vi "main.vi"() -> ()   [LabVIEW 2022 SP3]
uses:
  controls/State_control.ctl
  controls/Data.ctl
  <vilib>/Analysis/baseanly.llb/Mean (DBL).vi
  <vilib>/Utility/TDMS File Viewer/NI_TDMS File Viewer.lvlib
  <vilib>/Analysis/NI_AALBase.lvlib
panel:
  out "Prumerna teplota":dbl(graph)=53.18446
  out "Rozsah error":bool=TRUE
  out "Real-Time mereni":string[][](table)
  out "Prumerovane hodnoty":string[][](table)
  in  "vzorky/s":enum16{"Slow - 0.25 vz/s", "Fast - 12 vz/s"}(ring)=enum."Fast - 12 vz/s"
  in  "Pocet vz.":u16=20
  in  "Prumerovani":u16=10 min=1 max=20 step=1
  in  "Stop":bool
  in  "Koeficient termistoru [1/°C]":dbl=0.00385
  in  "Nazev souboru .tdms":path
  out "IDN Agilent 34450A":string
  out "Proud":dbl(graph)=0.489824809
  out "Napeti":dbl(graph)=53.18446
  out "IDN GPD-3303S":string
  in  "GPD-3303S":refnum<visa-resource-name>="zdroj"
  in  "Konec":bool
  in  "Start meas":bool
  out "IDN Agilent 34401A":string
  in  "Agilent 34401A":refnum<visa-resource-name>="01A"
  in  "Agilent 34450A":refnum<visa-resource-name>="50A"
  out "Stav":T1
  out "Ramecek":bool
  # "Kanaly"
  # "Parametry mereni"
  # "Uzivateli je doporuceno hodnoty zaokrouhlit podle platych pravidel"
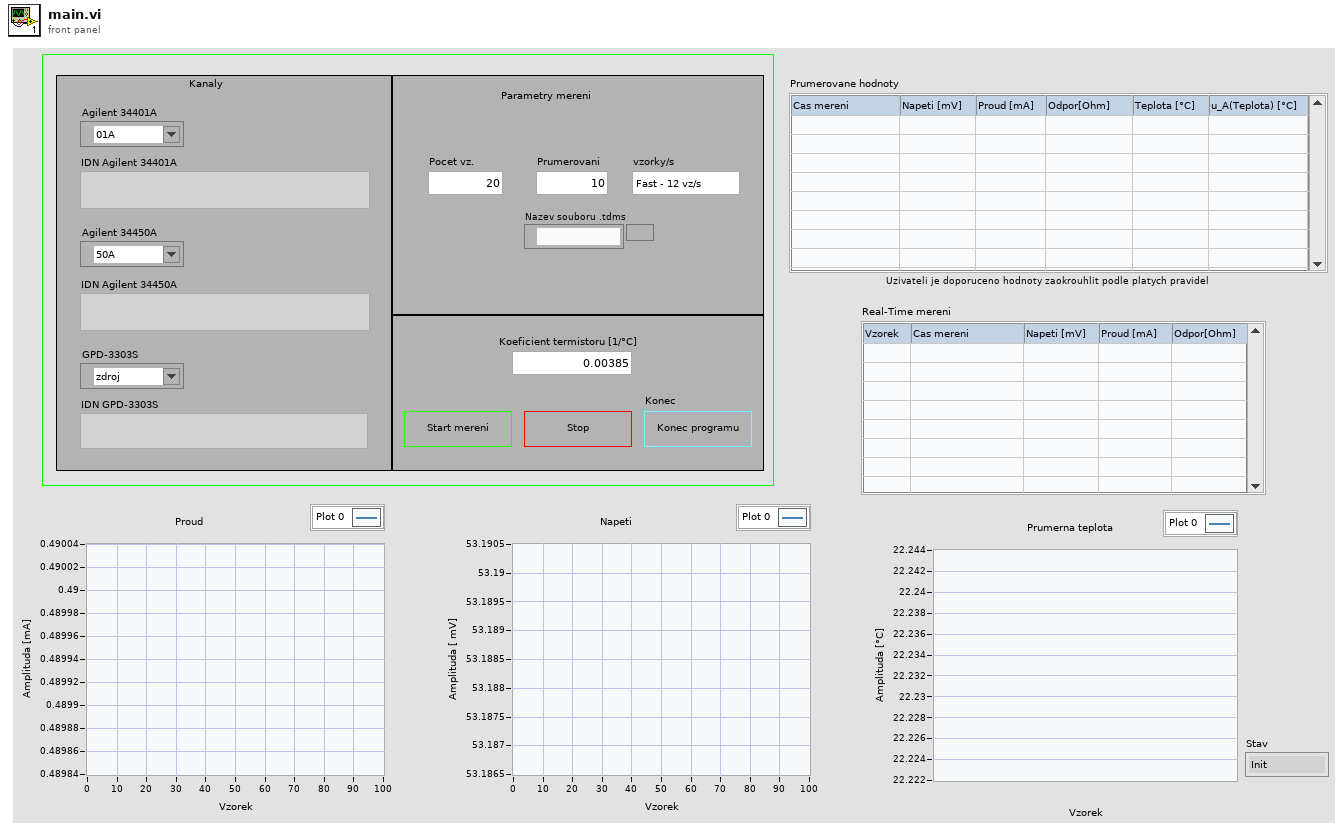
[diagram p1: front panel]
types:
  T1 = typedef "State_control.ctl" = enum16{"Init", "Waiting", "Measure", "SaveData", "Finish"}
  T2 = typedef "Data.ctl" = cluster{"No Sample":u16, "Samples/s":u16, "No to avg":u16, "Voltage":dbl[], "Current":dbl[], "Resistance":dbl[], "Temperature":dbl[], "Avg Voltage":dbl[], "Timestamp":timestamp[], "Avg Current":dbl[], "tdms file":refnum<k34>, "Timestamp avg":timestamp[], "Avg Resistance":dbl[], "Avg Temperature":dbl[], "u_A(temp)":dbl[]}
  T3 = enum8{"Enabled", "Disabled", "Disabled and Grayed Out"}
  T4 = enum16{"open", "open or create", "create or replace", "create", "open (read-only)"}
  T5 = cluster{"Agilent 34401A":refnum<visa-resource-name>, "Agilent 34450A":refnum<visa-resource-name>}
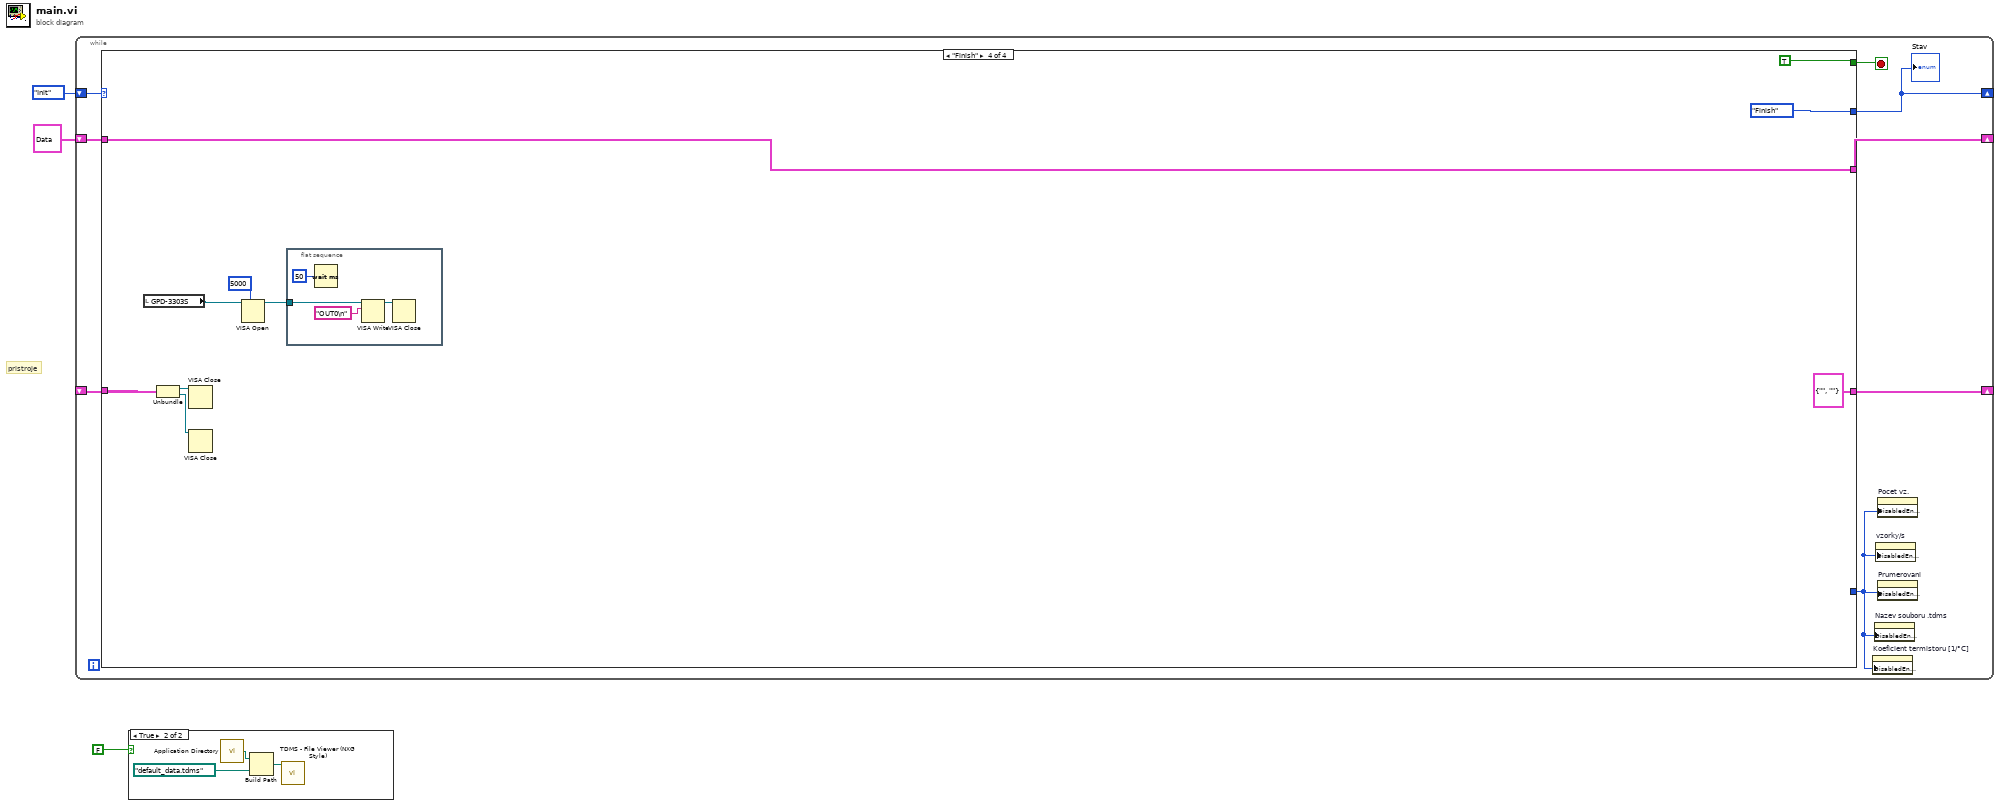
[diagram p0: block diagram]
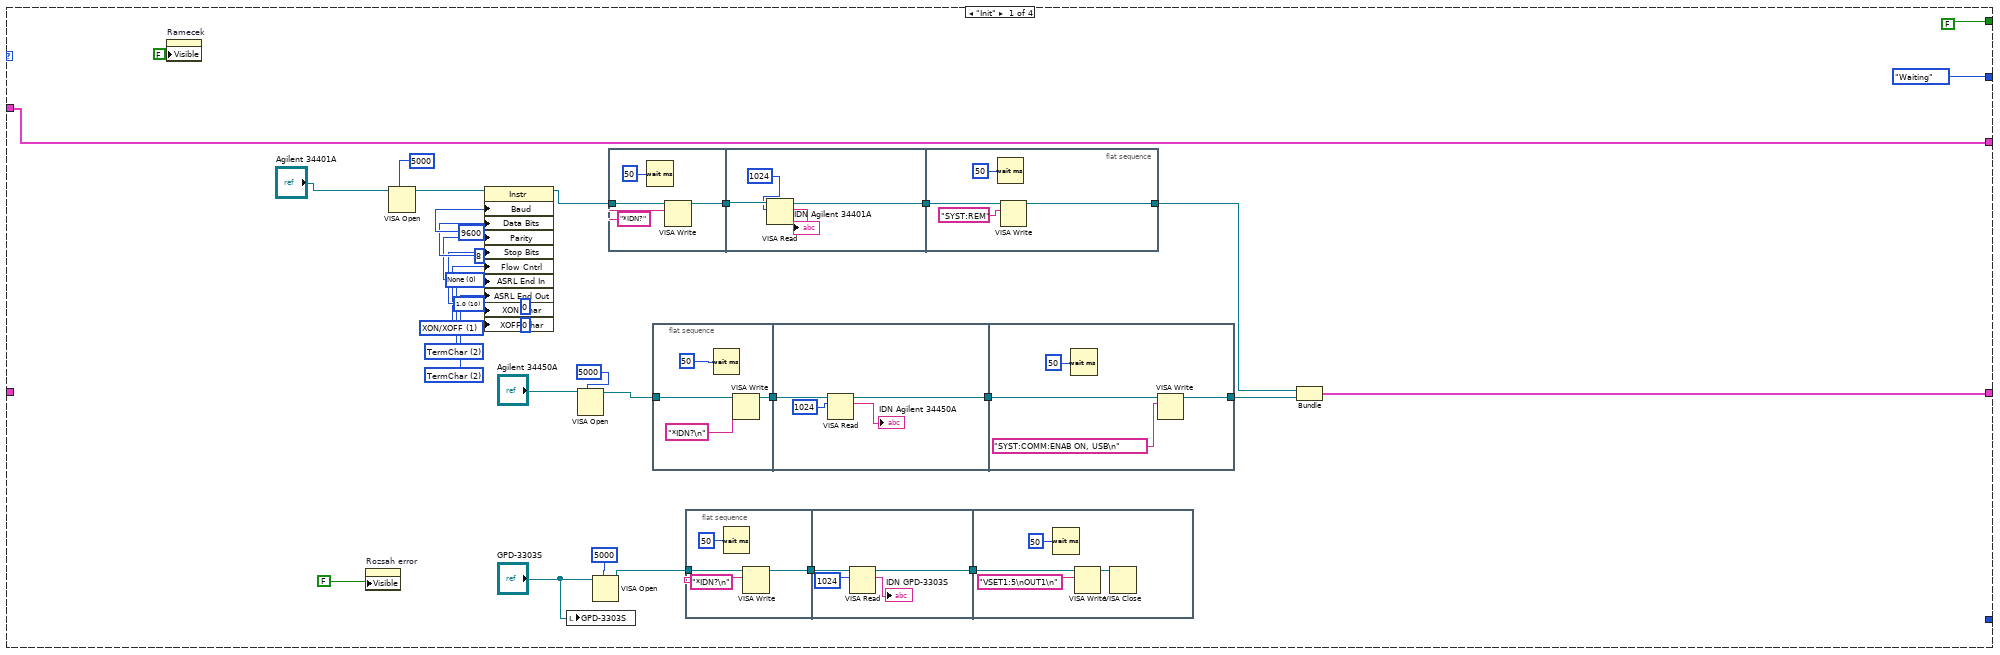
[diagram p2: hidden frame]
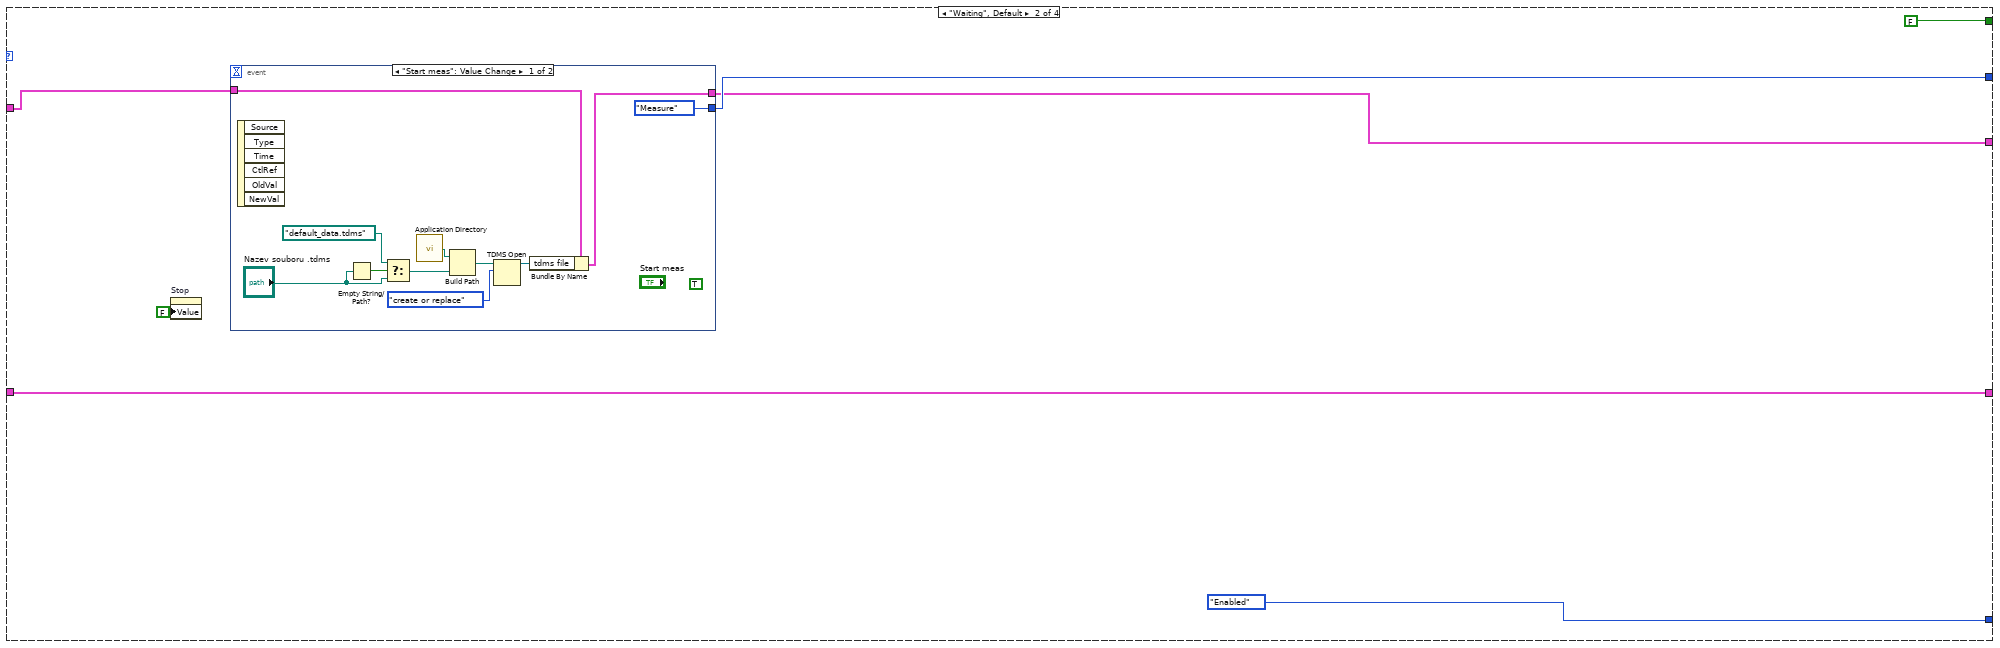
[diagram p3: hidden frame]
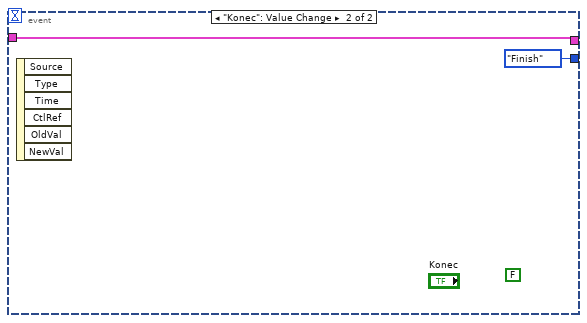
[diagram p4: hidden frame]
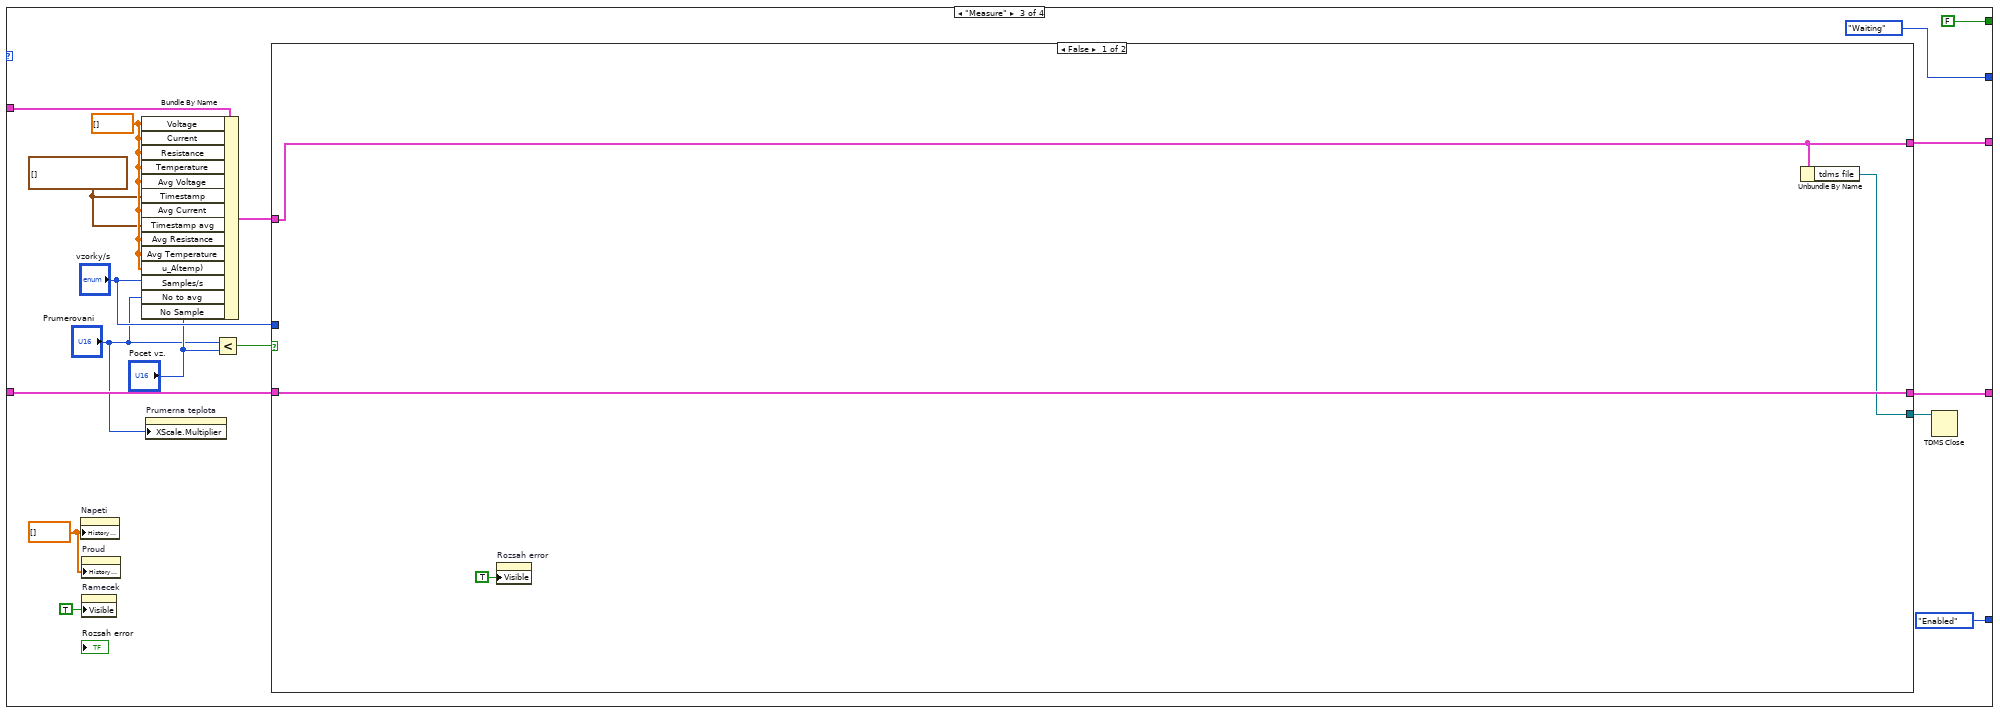
[diagram p5: hidden frame]
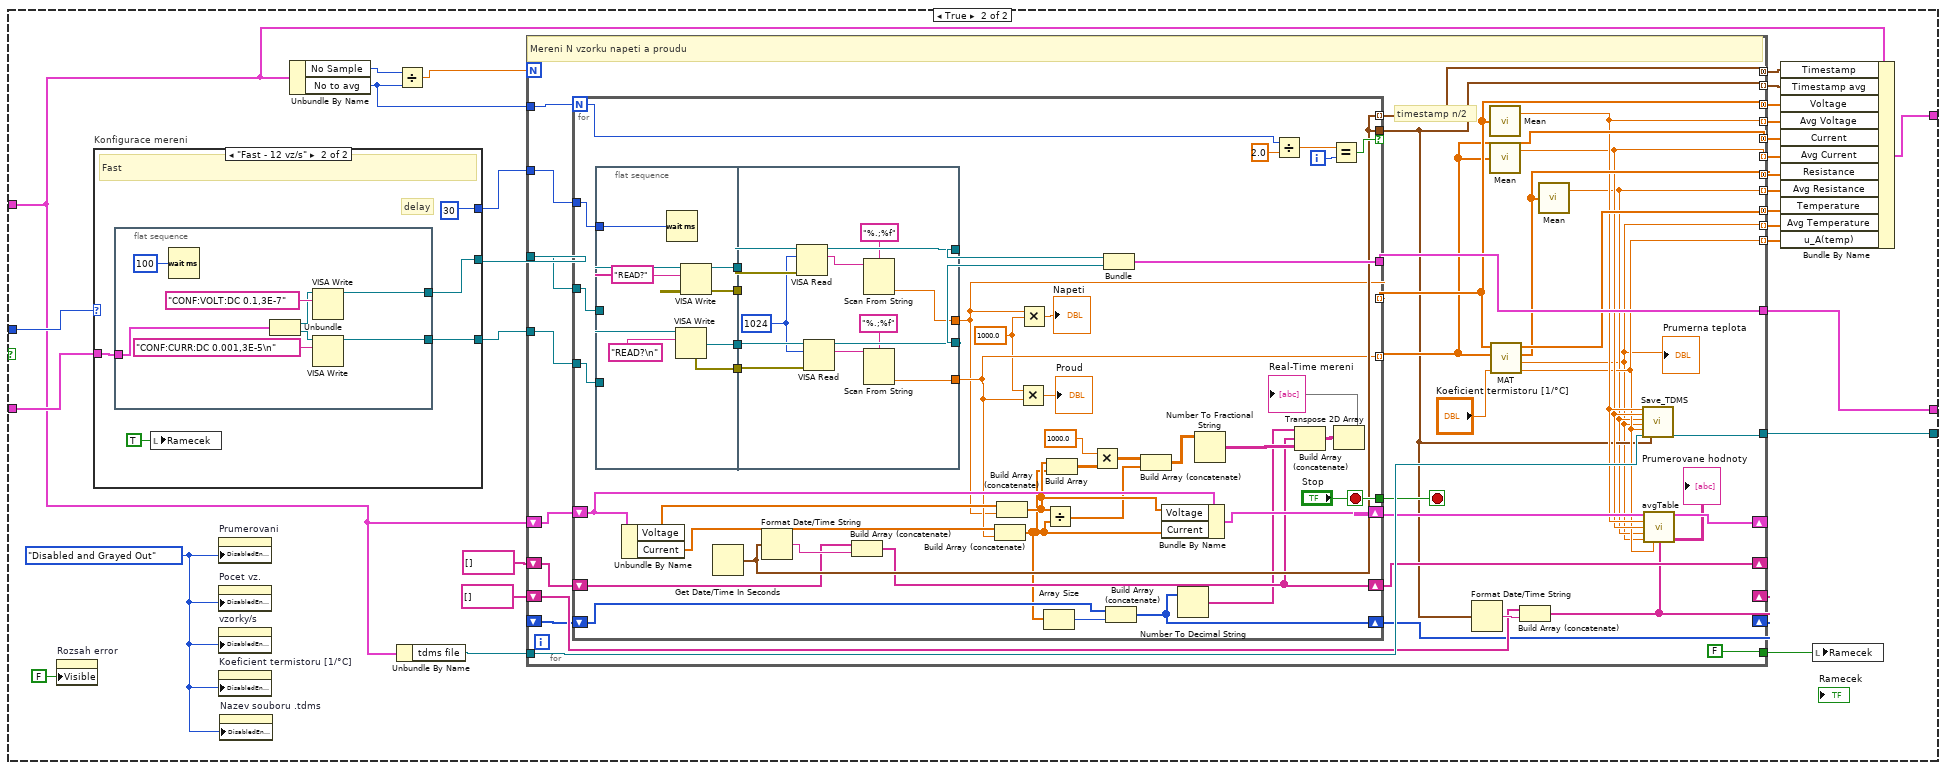
[diagram p6: hidden frame]
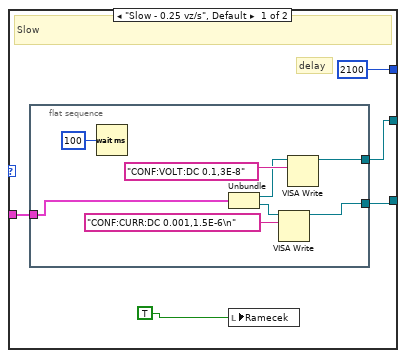
[diagram p7: hidden frame]
diagram:
  # "pristroje"
  n1 = while {
    shift-right: [w7] -> _
    shift-left: State_control."Init" ("State") -> [w11]
    shift-right: [w6] -> _
    shift-left: T2 {"No Sample"=0, "Samples/s"=0, "No to avg"=0, "Voltage"=[], "Current"=[], "Resistance"=[], "Temperature"=[], "Avg Voltage"=[], "Timestamp"=[], "Avg Current"=[], "tdms file"=refnum, "Timestamp avg"=[], "Avg Resistance"=[], "Avg Temperature"=[], "u_A(temp)"=[]} ("Data") -> [w5]
    shift-right: [w9] -> _
    shift-left: _ -> [w8]
    stop <- w10 stop-if-true
    n2 = case shown="\"Finish\"" w11 {
      tunnel: [State_control."Waiting" ("State 2") w85 State_control."Waiting" ("State 2") State_control."Finish" ("State 2")] -> w7
      tunnel: [FALSE FALSE FALSE TRUE] -> w10
      tunnel: w5 -> [w15 w83 w113 w278]
      tunnel: [w15 w82 w114 w278] -> w6
      tunnel: [w16 w86 w115 T5 {"Agilent 34401A"="", "Agilent 34450A"=""}] -> w9
      tunnel: w8 -> [_ w86 w116 w281]
      tunnel: [_ T3."Enabled" ("Disabled") T3."Enabled" ("Disabled") _] -> w4
      frame "Init" {
        w34 = u16 2 items=["None", "Last Bit", "TermChar", "Break"] ("Serial Settings:End Mode for Writes")
        w35 = u16 2 items=["None", "Last Bit", "TermChar"] ("Serial Settings:End Mode for Reads")
        w36 = u16 1 items=["None", "XON/XOFF", "RTS/CTS", "XON/XOFF & RTS/CTS", "DTR/DSR", "XON/XOFF & DTR/DSR"] ("Serial Settings:Flow Control")
        w37 = u16 10 items=["1.0"=10, "1.5"=15, "2.0"=20] ("Serial Settings:Stop Bits")
        w38 = u16 0 items=["None", "Odd", "Even", "Mark", "Space"] ("Serial Settings:Parity")
        n3 = property on="Ramecek" class="Bool (strict)"("Visible"=FALSE) -> ()  [unwired: 2 in, 2 out]
        n4 = property on="Rozsah error" class="Bool"("Visible"=FALSE) -> ()  [unwired: 2 in, 2 out]
        n5 = VISA Open(timeout (0)=u32 5000 ("VISA Open timeout (0)"), VISA resource name="Agilent 34401A") -> (VISA resource name=w41:refnum<visa-resource-name>)  [unwired: 3 in, 1 out]
        n6 = property class="Instr"(reference=w41, "Baud"=u32 9600 ("Serial Settings:Baud Rate"), "Data Bits"=u16 8 ("Serial Settings:Data Bits"), "Parity"=w38, "Stop Bits"=w37, "Flow Cntrl"=w36, "ASRL End In"=w35, "ASRL End Out"=w34, "XON Char"=u8 0 ("Serial Settings:Flow Control XON Character"), "XOFF Char"=u8 0 ("Serial Settings:Flow Control XOFF Character")) -> (reference out=w30:refnum<visa-resource-name>)  [unwired: 1 in, 1 out]
        n7 = local write "GPD-3303S"("GPD-3303S") -> ()
        n8 = VISA Open(timeout (0)=u32 5000 ("VISA Open timeout (0)"), VISA resource name="Agilent 34450A") -> (VISA resource name=w23:refnum<visa-resource-name>)  [unwired: 3 in, 1 out]
        n9 = VISA Open(timeout (0)=u32 5000 ("VISA Open timeout (0)"), VISA resource name="GPD-3303S") -> (VISA resource name=w19:refnum<visa-resource-name>)  [unwired: 3 in, 1 out]
        n10 = flat-sequence {
          tunnel: w30 -> [w72]
          tunnel: [w70] -> w31
          tunnel: w31 -> [w76]
          tunnel: [w75] -> w29
          tunnel: [w78] -> w18
          tunnel: w29 -> [w79]
          frame #0 {
            n11 = Wait (ms)(milliseconds to wait=u32 50) -> ()  [unwired: 1 out]
            n12 = VISA Write(VISA resource name=w72, write buffer="*IDN?") -> (VISA resource name out=w70:refnum<visa-resource-name>)  [unwired: 1 in, 2 out]
          }
          frame #1 {
            n13 = VISA Read(VISA resource name=w76, byte count=u32 1024) -> (VISA resource name out=w75:refnum<visa-resource-name>, read buffer=→"IDN Agilent 34401A":string)  [unwired: 1 in, 2 out]
          }
          frame #2 {
            n14 = Wait (ms)(milliseconds to wait=u32 50) -> ()  [unwired: 1 out]
            n15 = VISA Write(VISA resource name=w79, write buffer="SYST:REM") -> (VISA resource name out=w78:refnum<visa-resource-name>)  [unwired: 1 in, 2 out]
          }
        }
        n16 = flat-sequence {
          tunnel: [w59] -> w27
          tunnel: w23 -> [w57]
          tunnel: w27 -> [w63]
          tunnel: [w62] -> w26
          tunnel: [w65] -> w17
          tunnel: w26 -> [w66]
          frame #0 {
            n17 = Wait (ms)(milliseconds to wait=u32 50) -> ()  [unwired: 1 out]
            n18 = VISA Write(VISA resource name=w57, write buffer="*IDN?\n") -> (VISA resource name out=w59:refnum<visa-resource-name>)  [unwired: 1 in, 2 out]
          }
          frame #1 {
            n19 = VISA Read(VISA resource name=w63, byte count=u32 1024) -> (VISA resource name out=w62:refnum<visa-resource-name>, read buffer=→"IDN Agilent 34450A":string)  [unwired: 1 in, 2 out]
          }
          frame #2 {
            n20 = Wait (ms)(milliseconds to wait=u32 50) -> ()  [unwired: 1 out]
            n21 = VISA Write(VISA resource name=w66, write buffer="SYST:COMM:ENAB ON, USB\n") -> (VISA resource name out=w65:refnum<visa-resource-name>)  [unwired: 1 in, 2 out]
          }
        }
        n22 = flat-sequence {
          tunnel: [w47] -> w21
          tunnel: w19 -> [w45]
          tunnel: w21 -> [w51]
          tunnel: [w50] -> w20
          tunnel: w20 -> [w54]
          frame #0 {
            n23 = Wait (ms)(milliseconds to wait=u32 50) -> ()  [unwired: 1 out]
            n24 = VISA Write(VISA resource name=w45, write buffer="*IDN?\n") -> (VISA resource name out=w47:refnum<visa-resource-name>)  [unwired: 1 in, 2 out]
          }
          frame #1 {
            n25 = VISA Read(VISA resource name=w51, byte count=u32 1024) -> (VISA resource name out=w50:refnum<visa-resource-name>, read buffer=→"IDN GPD-3303S":string)  [unwired: 1 in, 2 out]
          }
          frame #2 {
            n26 = Wait (ms)(milliseconds to wait=u32 50) -> ()  [unwired: 1 out]
            n27 = VISA Write(VISA resource name=w54, write buffer="VSET1:5\nOUT1\n") -> (VISA resource name out=w53:refnum<visa-resource-name>)  [unwired: 1 in, 2 out]
            n28 = VISA Close(VISA resource name=w53) -> ()  [unwired: 1 in, 1 out]
          }
        }
        n29 = Bundle("Agilent 34401A"=w18, "Agilent 34450A"=w17) -> (w16:T5)  [unwired: 1 in]
      }
      frame "Waiting", Default {
        n30 = property on="Stop" class="Bool (strict)"("Value"=FALSE ("Stop")) -> ()  [unwired: 2 in, 2 out]
        n31 = event shown="[0] \"Start meas\": Value Change" {
          selector: _ -> [_ _]
          dyn-events: _ -> [_ _]
          timeout: _ -> [_ _]
          tunnel: [State_control."Measure" ("State 2") State_control."Finish" ("State 2")] -> w85
          tunnel: w83 -> [w89 w99]
          tunnel: [w88 w99] -> w82
          event "Start meas": Value Change {
            (unwired) TRUE
            n32 = event-data() -> ()  [unwired: 1 in, 6 out]
            n33 = Empty String/Path?(string/path="Nazev souboru .tdms") -> (empty?=w95:bool)
            n34 = Select(t=path "default_data.tdms", s=w95, f="Nazev souboru .tdms") -> (s? t:f=w93:path)
            n35 = call <vilib>:"Application Directory.vi"() -> ("Application Directory"=w97:path)
            n36 = Build Path(base path=w97, name or relative path=w93) -> (appended path=w96:path)
            n37 = TDMS Open(10:T4."create or replace" ("operation (0:open)"), 11:w96) -> (3:w90:refnum<k34>)  [unwired: 5 in, 1 out]
            n38 = Bundle By Name(cluster=w89, "tdms file"=w90) -> (w88:T2)
          }
          event "Konec": Value Change {
            (unwired) FALSE
            n39 = event-data() -> ()  [unwired: 1 in, 6 out]
          }
        }
      }
      frame "Measure" {
        w108 = dbl[] [] ("History Data")
        w111 = timestamp[] [] ("Timestamp")
        w112 = dbl[] [] ("Voltage")
        n40 = property on="Napeti" class="WFChart (strict)"("History Data"=w108) -> ()  [unwired: 2 in, 2 out]
        n41 = property on="Proud" class="WFChart (strict)"("History Data"=w108) -> ()  [unwired: 2 in, 2 out]
        n42 = property on="Ramecek" class="Bool (strict)"("Visible"=TRUE) -> ()  [unwired: 2 in, 2 out]
        n43 = Bundle By Name(cluster=w113, "Voltage"=w112, "Current"=w112, "Resistance"=w112, "Temperature"=w112, "Avg Voltage"=w112, "Timestamp"=w111, "Avg Current"=w112, "Timestamp avg"=w111, "Avg Resistance"=w112, "Avg Temperature"=w112, "u_A(temp)"=w112, "Samples/s"="vzorky/s", "No to avg"="Prumerovani", "No Sample"="Pocet vz.") -> (w110:T2)
        n44 = property on="Prumerna teplota" class="WFChart (strict)"("XScale.Multiplier"="Prumerovani") -> ()  [unwired: 2 in, 2 out]
        n45 = Less?(x="Prumerovani", y="Pocet vz.") -> (x < y?=w105:bool)
        n46 = case shown="False" w105 {
          tunnel: w116 -> [w121 w150]
          tunnel: [w121 w146] -> w115
          tunnel: [w118 w143] -> w114
          tunnel: w110 -> [w118 w122]
          tunnel: "vzorky/s" -> [_ w127]
          tunnel: [w120 w125] -> w104
          frame False {
            n47 = property on="Rozsah error" class="Bool"("Visible"=TRUE) -> ()  [unwired: 2 in, 2 out]
            n48 = Unbundle By Name(w118) -> ("tdms file"=w120:refnum<k34>)
          }
          frame True {
            w130 = T3."Disabled and Grayed Out" ("Disabled")
            n49 = property on="Rozsah error" class="Bool"("Visible"=FALSE) -> ()  [unwired: 2 in, 2 out]
            n50 = case "Konfigurace mereni" shown="\"Fast - 12 vz/s\"" w127 {
              tunnel: w150 -> [w252 w265]
              tunnel: [w249 w264] -> w149
              tunnel: [w250 w263] -> w148
              tunnel: [u32 2100 ("milliseconds to wait") u32 30 ("milliseconds to wait")] -> w147
              frame "Slow - 0.25 vz/s", Default {
                # "delay"
                # "Slow"
                n51 = flat-sequence {
                  tunnel: [w258] -> w250
                  tunnel: w252 -> [w255]
                  tunnel: [w257] -> w249
                  frame #0 {
                    n52 = Wait (ms)(milliseconds to wait=u32 100) -> ()  [unwired: 1 out]
                    n53 = Unbundle(w255) -> ("Agilent 34401A"=w254:refnum<visa-resource-name>, "Agilent 34450A"=w253:refnum<visa-resource-name>)
                    n54 = VISA Write(VISA resource name=w253, write buffer="CONF:CURR:DC 0.001,1.5E-6\n") -> (VISA resource name out=w257:refnum<visa-resource-name>)  [unwired: 1 in, 2 out]
                    n55 = VISA Write(VISA resource name=w254, write buffer="CONF:VOLT:DC 0.1,3E-8") -> (VISA resource name out=w258:refnum<visa-resource-name>)  [unwired: 1 in, 2 out]
                  }
                }
                n56 = local write "Ramecek"(TRUE ("Ramecek")) -> ()
              }
              frame "Fast - 12 vz/s" {
                # "delay"
                # "Fast"
                n57 = flat-sequence {
                  tunnel: [w271] -> w263
                  tunnel: w265 -> [w268]
                  tunnel: [w270] -> w264
                  frame #0 {
                    n58 = Wait (ms)(milliseconds to wait=u32 100) -> ()  [unwired: 1 out]
                    n59 = Unbundle(w268) -> ("Agilent 34401A"=w267:refnum<visa-resource-name>, "Agilent 34450A"=w266:refnum<visa-resource-name>)
                    n60 = VISA Write(VISA resource name=w267, write buffer="CONF:VOLT:DC 0.1,3E-7") -> (VISA resource name out=w271:refnum<visa-resource-name>)  [unwired: 1 in, 2 out]
                    n61 = VISA Write(VISA resource name=w266, write buffer="CONF:CURR:DC 0.001,3E-5\n") -> (VISA resource name out=w270:refnum<visa-resource-name>)  [unwired: 1 in, 2 out]
                  }
                }
                n62 = local write "Ramecek"(TRUE ("Ramecek")) -> ()
              }
            }
            n63 = property on="Prumerovani" class="DigNum (strict)"("DisabledEnum"=w130) -> ()  [unwired: 2 in, 2 out]
            n64 = property on="Pocet vz." class="DigNum (strict)"("DisabledEnum"=w130) -> ()  [unwired: 2 in, 2 out]
            n65 = property on="vzorky/s" class="Enum (strict)"("DisabledEnum"=w130) -> ()  [unwired: 2 in, 2 out]
            n66 = property on="Koeficient termistoru [1/°C]" class="DigNum (strict)"("DisabledEnum"=w130) -> ()  [unwired: 2 in, 2 out]
            n67 = property on="Nazev souboru .tdms" class="Path"("DisabledEnum"=w130) -> ()  [unwired: 2 in, 2 out]
            n68 = Unbundle By Name(w122) -> ("No Sample"=w123:u16, "No to avg"=w144:u16)
            n69 = Divide(x=w123, y=w144) -> (x/y=w145:dbl)
            n70 = Unbundle By Name(w122) -> ("tdms file"=w131:refnum<k34>)
            n71 = for {
              N: w145 -> [_]
              tunnel: w149 -> [w182]
              tunnel: w148 -> [w181]
              tunnel: [w180] -> w146
              tunnel: w147 -> [w179]
              tunnel: w144 -> [w175]
              tunnel: [w178] -> w138 mode=concatenating
              tunnel: [w174] -> w142 mode=concatenating
              tunnel: [w173] -> w141 mode=concatenating
              tunnel: [w172] -> w140 mode=concatenating
              tunnel: [w176] -> w139 mode=concatenating
              tunnel: [w160] -> w137 mode=indexing
              tunnel: [w151] -> w136 mode=indexing
              tunnel: [w161] -> w135 mode=indexing
              tunnel: [w163] -> w134 mode=indexing
              tunnel: [w162] -> w133 mode=indexing
              tunnel: [w152] -> w132 mode=indexing
              tunnel: w131 -> [w171]
              tunnel: [w170] -> w125
              shift-right: [w164] -> _
              shift-left: w122 -> [w168]
              shift-right: [w167] -> _
              shift-left: string[] [] -> [w166]
              shift-right: [w156] -> _
              shift-left: string[] [] -> [w158]
              shift-right: [w155] -> _
              shift-left: _ -> [w154]
              tunnel: [FALSE ("Ramecek")] -> w126
              stop <- w169 stop-if-true
              # "timestamp n/2"
              # "Mereni N vzorku napeti a proudu"
              n72 = for {
                N: w175 -> [w211]
                tunnel: w182 -> [w221]
                tunnel: w181 -> [w220]
                tunnel: [w217] -> w180
                tunnel: w179 -> [w216]
                tunnel: [w204] -> w178 mode=indexing
                tunnel: [w195] -> w174 mode=indexing
                tunnel: [w198] -> w173 mode=indexing
                tunnel: [w204] -> w160 if=w215
                tunnel: ["Stop"] -> w169
                shift-right: [w209] -> w165
                shift-left: w168 -> [w208]
                shift-right: [w201] -> w167
                shift-left: w166 -> [w202]
                shift-right: [w191] -> w155
                shift-left: w154 -> [w193]
                i -> [w214]
                stop <- "Stop" stop-if-true
                w194 = 1000.0
                n73 = flat-sequence {
                  tunnel: [w234] -> w225
                  tunnel: w220 -> [w233]
                  tunnel: [w232] -> w224
                  tunnel: w221 -> [w231]
                  tunnel: [w230] -> w223
                  tunnel: [w229] -> w222
                  tunnel: w216 -> [w226]
                  tunnel: w225 -> [w246]
                  tunnel: [w247] -> w219
                  tunnel: w224 -> [w245]
                  tunnel: w223 -> [w244]
                  tunnel: w222 -> [w243]
                  tunnel: [w242] -> w218
                  tunnel: [w239] -> w195
                  tunnel: [w235] -> w198
                  frame #0 {
                    n74 = Wait (ms)(milliseconds to wait=w226) -> ()  [unwired: 1 out]
                    n75 = VISA Write(VISA resource name=w231, write buffer="READ?\n") -> (VISA resource name out=w229:refnum<visa-resource-name>, error out=w230:errorcluster)  [unwired: 1 in, 1 out]
                    n76 = VISA Write(VISA resource name=w233, write buffer="READ?") -> (VISA resource name out=w234:refnum<visa-resource-name>, error out=w232:errorcluster)  [unwired: 1 in, 1 out]
                  }
                  frame #1 {
                    w241 = u32 1024 ("byte count")
                    n77 = VISA Read(VISA resource name=w246, byte count=w241, error in (no error)=w245) -> (VISA resource name out=w247:refnum<visa-resource-name>, read buffer=w240:string)  [unwired: 2 out]
                    n78 = VISA Read(VISA resource name=w243, byte count=w241, error in (no error)=w244) -> (VISA resource name out=w242:refnum<visa-resource-name>, read buffer=w238:string)  [unwired: 2 out]
                    n79 = Scan From String(format string="%.;%f", input string=w240) -> (output 1=w239:dbl)  [unwired: 3 in, 3 out]
                    n80 = Scan From String(format string="%.;%f", input string=w238) -> (output 1=w235:dbl)  [unwired: 3 in, 3 out]
                  }
                }
                n81 = Unbundle By Name(w208) -> ("Voltage"=w207:dbl[], "Current"=w206:dbl[])
                n82 = Get Date/Time In Seconds() -> (seconds since 1Jan1904=w204:timestamp)
                n83 = Format Date/Time String(seconds (now)=w204) -> (date/time string=w203:string)  [unwired: 2 in]
                n84 = Build Array (concatenate)(w202, w203) -> (w201:string[])
                n85 = Build Array (concatenate)(w206, w198) -> (w188:dbl[])
                n86 = Build Array (concatenate)(w207, w195) -> (w189:dbl[])
                n87 = Multiply(x=w194, y=w198) -> (x*y=→"Proud":dbl)
                n88 = Multiply(x=w195, y=w194) -> (x*y=→"Napeti":dbl)
                n89 = Array Size(array=w188) -> (size(s)=w192:i32)
                n90 = Divide(x=w189, y=w188) -> (x/y=w183:dbl[])
                n91 = Build Array(w189, w188) -> (w186:dbl[][])
                n92 = Multiply(x=1000.0, y=w186) -> (x*y=w185:dbl[][])
                n93 = Bundle("Agilent 34401A"=w219, "Agilent 34450A"=w218) -> (w217:T5)  [unwired: 1 in]
                n94 = Build Array (concatenate)(w193, w192) -> (w191:i32[])
                n95 = Build Array (concatenate)(w185, w183) -> (w184:dbl[][])
                n96 = Bundle By Name(cluster=w208, "Voltage"=w189, "Current"=w188) -> (w209:T2)
                n97 = Number To Decimal String(number=w191) -> (decimal integer string=w190:string[])  [unwired: 1 in]
                n98 = Number To Fractional String(number=w184) -> (F-format string=w205:string[][])  [unwired: 3 in]
                n99 = Divide(x=w211, y=2.0) -> (x/y=w212:dbl)
                n100 = Build Array (concatenate)(w190, w201, w205) -> (w200:string[][])
                n101 = Equal?(x=w212, y=w214) -> (x = y?=w215:bool)
                n102 = Transpose 2D Array(2D array=w200) -> (transposed array=→"Real-Time mereni":string[][])
              }
              n103 = Format Date/Time String(seconds (now)=w160) -> (date/time string=w159:string)  [unwired: 2 in]
              n104 = call-poly <vilib>:"Mean.vi"("X"=w174) -> ("mean"=w163:dbl)  [unwired: 1 out]
              n105 = call-poly <vilib>:"Mean.vi"("X"=w173) -> ("mean"=w162:dbl)  [unwired: 1 out]
              n106 = call "MAT.vi"("Alfa term"="Koeficient termistoru [1/°C]", "Current"=w173, "Voltage"=w174) -> ("u_A"=w161:dbl, "avg_temp"=w151:dbl, "Resistance"=w172:dbl[], "Temp"=w176:dbl[])  [unwired: 5 in]
              "Prumerna teplota" <- w151
              n107 = Build Array (concatenate)(w158, w159) -> (w156:string[])
              n108 = call-poly <vilib>:"Mean.vi"("X"=w172) -> ("mean"=w152:dbl)  [unwired: 1 out]
              n109 = call "Save_TDMS.vi"("Voltage"=w163, "Current"=w162, "Resistance"=w152, "Temperature"=w151, "u_A(temp)"=w161, "TDMS IN"=w171, "Timestamp"=w160) -> ("TDMS OUT"=w170:refnum<k34>)  [unwired: 12 in]
              n110 = call "avgTable.vi"("Data in"=w165, "Avg Voltage"=w163, "Avg Current"=w162, "Avg Resistance"=w152, "Avg Temperature"=w151, "u_A(temp)"=w161, "Timestamp string"=w156) -> ("Data out"=w164:T2, "Table"=→"Prumerovane hodnoty":string[][])  [unwired: 7 in]
            }
            n111 = Bundle By Name(cluster=w122, "Timestamp"=w138, "Timestamp avg"=w137, "Voltage"=w142, "Avg Voltage"=w134, "Current"=w141, "Avg Current"=w133, "Resistance"=w140, "Avg Resistance"=w132, "Temperature"=w139, "Avg Temperature"=w136, "u_A(temp)"=w135) -> (w143:T2)
            n112 = local write "Ramecek"(w126) -> ()
          }
        }
        n113 = TDMS Close(11:w104) -> ()  [unwired: 1 in, 2 out]
      }
      frame "Finish" {
        n114 = local read "GPD-3303S"() -> (w276:refnum<visa-resource-name>)
        n115 = Unbundle(w281) -> ("Agilent 34401A"=w280:refnum<visa-resource-name>, "Agilent 34450A"=w279:refnum<visa-resource-name>)
        n116 = VISA Close(VISA resource name=w280) -> ()  [unwired: 1 in, 1 out]
        n117 = VISA Close(VISA resource name=w279) -> ()  [unwired: 1 in, 1 out]
        n118 = VISA Open(timeout (0)=u32 5000 ("VISA Open timeout (0)"), VISA resource name=w276) -> (VISA resource name=w275:refnum<visa-resource-name>)  [unwired: 3 in, 1 out]
        n119 = flat-sequence {
          tunnel: w275 -> [w284]
          frame #0 {
            n120 = Wait (ms)(milliseconds to wait=u32 50) -> ()  [unwired: 1 out]
            n121 = VISA Write(VISA resource name=w284, write buffer="OUT0\n") -> (VISA resource name out=w285:refnum<visa-resource-name>)  [unwired: 1 in, 2 out]
            n122 = VISA Close(VISA resource name=w285) -> ()  [unwired: 1 in, 1 out]
          }
        }
      }
    }
    "Stav" <- w7
    n123 = property on="Koeficient termistoru [1/°C]" class="DigNum (strict)"("DisabledEnum"=w4) -> ()  [unwired: 2 in, 2 out]
    n124 = property on="Nazev souboru .tdms" class="Path"("DisabledEnum"=w4) -> ()  [unwired: 2 in, 2 out]
    n125 = property on="vzorky/s" class="Enum (strict)"("DisabledEnum"=w4) -> ()  [unwired: 2 in, 2 out]
    n126 = property on="Pocet vz." class="DigNum (strict)"("DisabledEnum"=w4) -> ()  [unwired: 2 in, 2 out]
    n127 = property on="Prumerovani" class="DigNum (strict)"("DisabledEnum"=w4) -> ()  [unwired: 2 in, 2 out]
  }
  n128 = case shown="True" FALSE {
    frame False {
    }
    frame True {
      n129 = call <vilib>:"Application Directory.vi"() -> ("Application Directory"=w290:path)
      n130 = Build Path(base path=w290, name or relative path=path "default_data.tdms") -> (appended path=w288:path)
      n131 = call <vilib>:"TDMS - File Viewer (NXG Style).vi"("file in"=w288) -> ()  [unwired: 9 in, 2 out]
    }
  }
